vi "ResultsTable (SubVI).vi"(8 "error in (no error)":errorcluster, 10 "Match Labels":string[](array[string]), 11 "Matches":T1[](array[typedef]) {"Correlation Score" format="%.2f"; "Target Template Curve Score" format="%.2f"; "Template Target Curve Score" format="%.2f"; "Bounding Box"."y" format="%.2f"; "Bounding Box"."x" format="%.2f"; "Position"."y" format="%.2f"; "Position"."x" format="%.2f"; "Score" format="%.2f"; "Scale" format="%.2f"; "Angle" format="%.2f"; "Occlusion %" format="%.2f"}) -> (0 "error out":errorcluster, 3 "Text Results":string[][](table))   [LabVIEW 2011]
uses:
  <vilib>/vision/Pattern Matching.llb/IMAQ GM Match Report.ctl
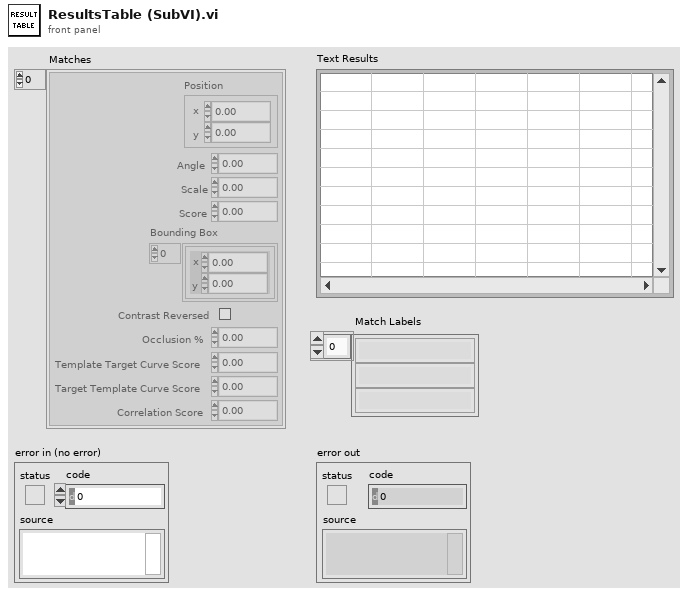
[diagram p1: front panel]
types:
  T1 = typedef "IMAQ GM Match Report.ctl" = cluster{"Position":cluster{"x":sgl, "y":sgl}, "Angle":sgl, "Scale":sgl, "Score":sgl, "Bounding Box":cluster{"x":sgl, "y":sgl}[], "Contrast Reversed":bool, "Occlusion %":sgl, "Template Target Curve Score":sgl, "Target Template Curve Score":sgl, "Correlation Score":sgl}
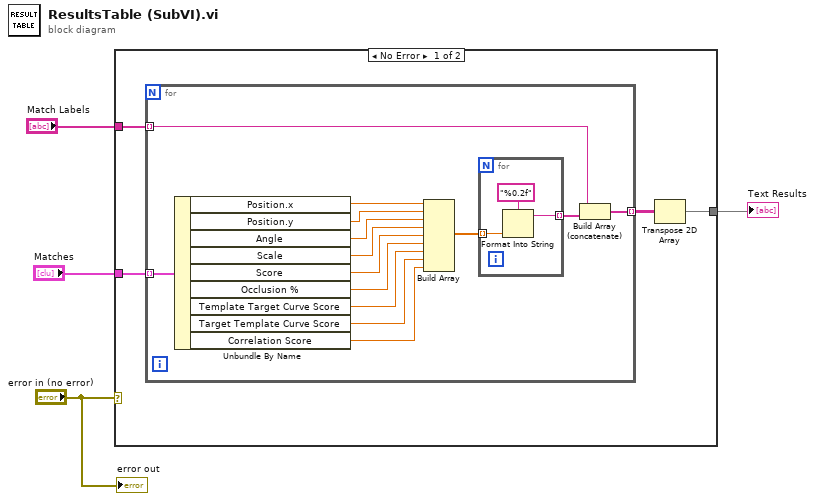
[diagram p0: block diagram]
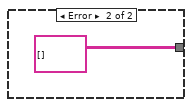
[diagram p2: hidden frame]
diagram:
  n1 = case shown="No Error" "error in (no error)" {
    tunnel: "Matches" -> [w8 _]
    tunnel: [w6 string[][] []] -> w3
    tunnel: "Match Labels" -> [w5 _]
    frame No Error {
      n2 = for {
        tunnel: w8 -> [w22] mode=indexing
        tunnel: [w10] -> w7 mode=indexing
        tunnel: w5 -> [w9] mode=indexing
        n3 = Unbundle By Name(w22) -> ("Position.x"=w21:sgl, "Position.y"=w20:sgl, "Angle"=w19:sgl, "Scale"=w18:sgl, "Score"=w17:sgl, "Occlusion %"=w16:sgl, "Template Target Curve Score"=w15:sgl, "Target Template Curve Score"=w14:sgl, "Correlation Score"=w13:sgl)
        n4 = Build Array(w21, w20, w19, w18, w17, w16, w15, w14, w13) -> (w12:sgl[])
        n5 = for {
          tunnel: w12 -> [w25] mode=indexing
          tunnel: [w23] -> w11 mode=indexing
          n6 = Format Into String(format string="%0.2f", w25) -> (resulting string=w23:string)  [unwired: 2 in, 1 out]
        }
        n7 = Build Array (concatenate)(w9, w11) -> (w10:string[])
      }
      n8 = Transpose 2D Array(2D array=w7) -> (transposed array=w6:string[][])
    }
    frame Error {
    }
  }
  "Text Results" <- w3
  "error out" <- "error in (no error)"
